vi "test_MSS SimulatedScope SimulatedFGen on ref in parallel.vi"(8 "Error In":errorcluster) -> (0 "Error Out":errorcluster)   [LabVIEW 2023]
uses:
  Measure and Stimulus Subsystems/Measure and Stimulus Subsystems.lvclass
panel:
  out "time":dbl
  out "Photosensor Waveform Chart":waveform(dbl)(graph)
  in  "Stop":bool
  out "Powersensor Scalar":dbl
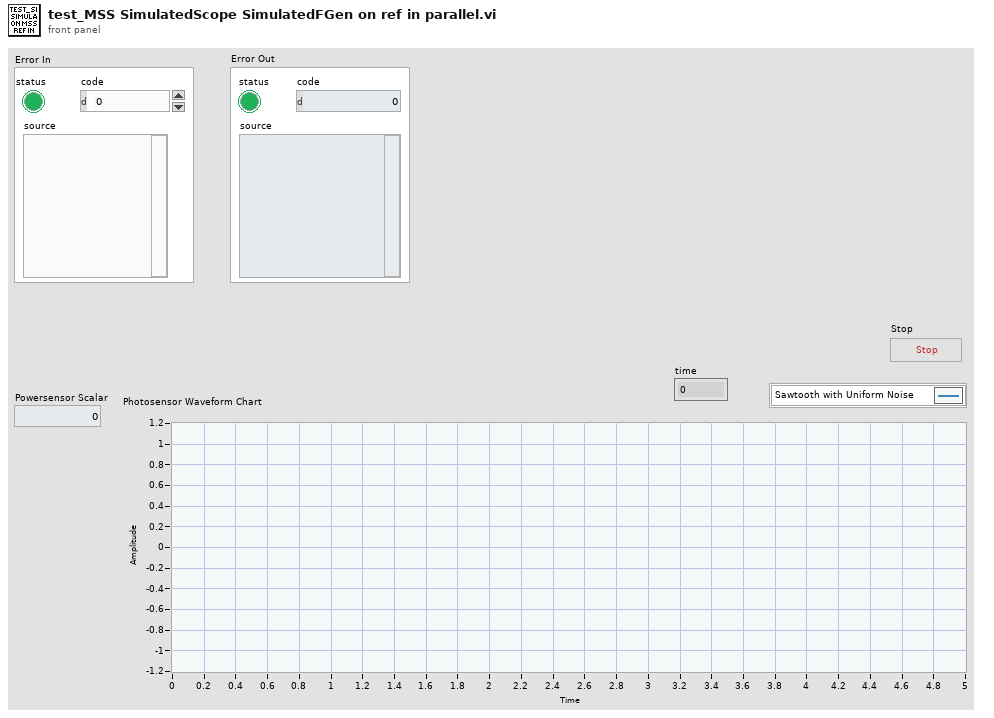
[diagram p1: front panel]
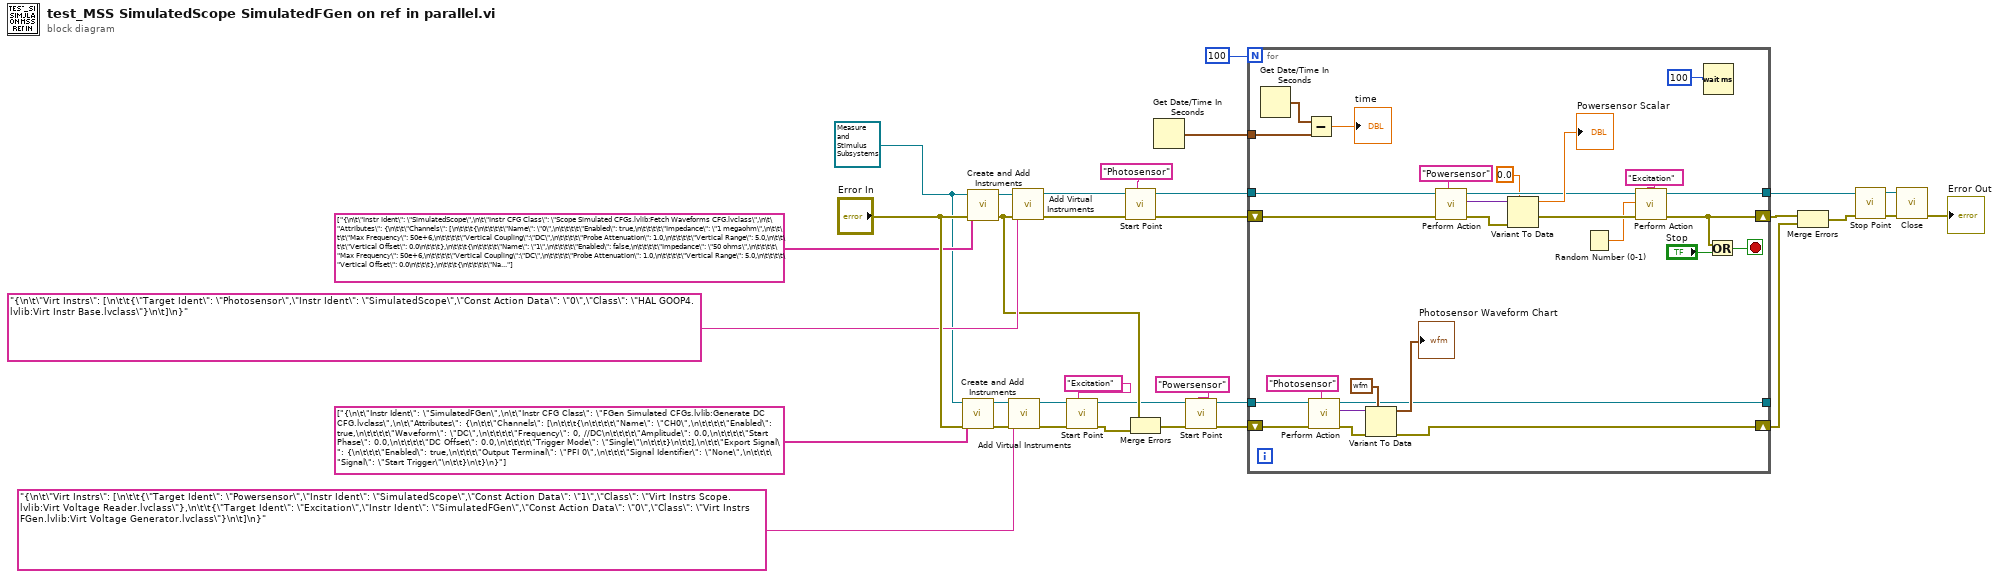
[diagram p0: block diagram]
diagram:
  w1 = refnum<class "Measure and Stimulus Subsystems.lvclass"> refnum ("MSS in")
  n1 = call "Create and Add Instruments.vi"("Error In"="Error In", "Physical Intr CFGs"=string[] ["{\n\t\"Instr Ident\": \"SimulatedFGen\",\n\t\"Instr CFG Class\": \"FGen Simulated CFGs.lvlib:Generate DC CFG.lvclass\",\n\t\"Attributes\": {\n\t\t\"Channels\": [\n\t\t\t{\n\t\t\t\t\"Name\": \"CH0\",\n\t\t\t\t\"Enabled\": true,\n\t\t\t\t\"Waveform\": \"DC\",\n\t\t\t\t\"Frequency\": 0, //DC\n\t\t\t\t\"Amplitude\": 0.0,\n\t\t\t\t\"Start Phase\": 0.0,\n\t\t\t\t\"DC Offset\": 0.0,\n\t\t\t\t\"Trigger Mode\": \"Single\"\n\t\t\t}\n\t\t],\n\t\t\"Export Signal\": {\n\t\t\t\"Enabled\": true,\n\t\t\t\"Output Terminal\": \"PFI 0\",\n\t\t\t\"Signal Identifier\": \"None\",\n\t\t\t\"Signal\": \"Start Trigger\"\n\t\t}\n\t}\n}"], "MSS in"=w1) -> ("Error Out"=w17:errorcluster, "MSS out"=w16:refnum<class "Measure and Stimulus Subsystems.lvclass">)  [unwired: 7 in]
  n2 = call "Create and Add Instruments.vi"("Error In"="Error In", "Physical Intr CFGs"=string[] ["{\n\t\"Instr Ident\": \"SimulatedScope\",\n\t\"Instr CFG Class\": \"Scope Simulated CFGs.lvlib:Fetch Waveforms CFG.lvclass\",\n\t\"Attributes\": {\n\t\t\"Channels\": [\n\t\t\t{\n\t\t\t\t\"Name\": \"0\",\n\t\t\t\t\"Enabled\": true,\n\t\t\t\t\"Impedance\": \"1 megaohm\",\n\t\t\t\t\"Max Frequency\": 50e+6,\n\t\t\t\t\"Vertical Coupling\":\"DC\",\n\t\t\t\t\"Probe Attenuation\": 1.0,\n\t\t\t\t\"Vertical Range\": 5.0,\n\t\t\t\t\"Vertical Offset\": 0.0\n\t\t\t},\n\t\t\t{\n\t\t\t\t\"Name\": \"1\",\n\t\t\t\t\"Enabled\": false,\n\t\t\t\t\"Impedance\": \"50 ohms\",\n\t\t\t\t\"Max Frequency\": 50e+6,\n\t\t\t\t\"Vertical Coupling\":\"DC\",\n\t\t\t\t\"Probe Attenuation\": 1.0,\n\t\t\t\t\"Vertical Range\": 5.0,\n\t\t\t\t\"Vertical Offset\": 0.0\n\t\t\t},\n\t\t\t{\n\t\t\t\t\"Name\": \"2\",\n\t\t\t\t\"Enabled\": false,\n\t\t\t\t\"Impedance\": \"50 ohms\",\n\t\t\t\t\"Max Frequency\": 50e+6,\n\t\t\t\t\"Vertical Coupling\":\"DC\",\n\t\t\t\t\"Probe Attenuation\": 1.0,\n\t\t\t\t\"Vertical Range\": 5.0,\n\t\t\t\t\"Vertical Offset\": 0.0\n\t\t\t},\n\t\t\t{\n\t\t\t\t\"Name\": \"3\",\n\t\t\t\t\"Enabled\": true,\n\t\t\t\t\"Impedance\": \"50 ohms\",\n\t\t\t\t\"Max Frequency\": 50e+6,\n\t\t\t\t\"Vertical Coupling\":\"DC\",\n\t\t\t\t\"Probe Attenuation\": 1.0,\n\t\t\t\t\"Vertical Range\": 1.4,\n\t\t\t\t\"Vertical Offset\": 0.0\n\t\t\t},\n\t\t\t{\n\t\t\t\t\"Name\": \"4\",\n\t\t\t\t\"Enabled\": false,\n\t\t\t\t\"Impedance\": \"50 ohms\",\n\t\t\t\t\"Max Frequency\": 50e+6,\n\t\t\t\t\"Vertical Coupling\":\"DC\",\n\t\t\t\t\"Probe Attenuation\": 1.0,\n\t\t\t\t\"Vertical Range\": 5.0,\n\t\t\t\t\"Vertical Offset\": 0.0\n\t\t\t},\n\t\t\t{\n\t\t\t\t\"Name\": \"5\",\n\t\t\t\t\"Enabled\": false,\n\t\t\t\t\"Impedance\": \"50 ohms\",\n\t\t\t\t\"Max Frequency\": 50e+6,\n\t\t\t\t\"Vertical Coupling\":\"DC\",\n\t\t\t\t\"Probe Attenuation\": 1.0,\n\t\t\t\t\"Vertical Range\": 5.0,\n\t\t\t\t\"Vertical Offset\": 0.0\n\t\t\t},\n\t\t\t{\n\t\t\t\t\"Name\": \"6\",\n\t\t\t\t\"Enabled\": false,\n\t\t\t\t\"Impedance\": \"50 ohms\",\n\t\t\t\t\"Max Frequency\": 50e+6,\n\t\t\t\t\"Vertical Coupling\":\"DC\",\n\t\t\t\t\"Probe Attenuation\": 1.0,\n\t\t\t\t\"Vertical Range\": 5.0,\n\t\t\t\t\"Vertical Offset\": 0.0\n\t\t\t},\n\t\t\t{\n\t\t\t\t\"Name\": \"7\",\n\t\t\t\t\"Enabled\": false,\n\t\t\t\t\"Impedance\": \"50 ohms\",\n\t\t\t\t\"Max Frequency\": 50e+6,\n\t\t\t\t\"Vertical Coupling\":\"DC\",\n\t\t\t\t\"Probe Attenuation\": 1.0,\n\t\t\t\t\"Vertical Range\": 5.0,\n\t\t\t\t\"Vertical Offset\": 0.0\n\t\t\t}\n\t\t],\n\t\t\"Horizontal\": {\n\t\t\t\"Enforce Realtime\": true,\n\t\t\t\"Number of Records\": 1,\n\t\t\t\"Min Sample Rate\": 1e+5,\n\t\t\t\"Reference Position\":50, //percent\n\t\t\t\"Min Record Length\":1e+3\n\t\t},\n\t\t\"Acquire\": {\n\t\t\t\"Type\": \"Normal\",\n\t\t\t\"NumSamples\": 1e+3,\n\t\t\t\"Fetch Relative To\": \"Read Pointer\"\n\t\t},\n\t\t\"Export Signal\": {\n\t\t\t\"Signal Identifier\": \"None\",\n\t\t\t\"Signal\": \"None\",\n\t\t\t\"Output Terminal\": \"None\"\n\t\t},\n\t\t\"Trigger\": {\n\t\t\t\"Type\": \"Immediate\",\n\t\t\t\"Slope\": \"Positive\",\n\t\t\t\"Source\": \"RTSI 0\",\n\t\t\t\"Holdoff\": 0.0,\n\t\t\t\"Delay\": 0.0\n\t\t}\n\t}\n}"], "MSS in"=w1) -> ("Error Out"=w9:errorcluster, "MSS out"=w21:refnum<class "Measure and Stimulus Subsystems.lvclass">)  [unwired: 7 in]
  n3 = call "Add Virtual Instruments.vi"("error in"=w17, "<JSON CFG>"="{\n\t\"Virt Instrs\": [\n\t\t{\"Target Ident\": \"Powersensor\",\"Instr Ident\": \"SimulatedScope\",\"Const Action Data\": \"1\",\"Class\": \"Virt Instrs Scope.lvlib:Virt Voltage Reader.lvclass\"},\n\t\t{\"Target Ident\": \"Excitation\",\"Instr Ident\": \"SimulatedFGen\",\"Const Action Data\": \"0\",\"Class\": \"Virt Instrs FGen.lvlib:Virt Voltage Generator.lvclass\"}\n\t]\n}", "MSS in"=w16) -> ("error out"=w11:errorcluster, "MSS out"=w12:refnum<class "Measure and Stimulus Subsystems.lvclass">)  [unwired: 7 in]
  n4 = call "Add Virtual Instruments.vi"("error in"=w9, "<JSON CFG>"="{\n\t\"Virt Instrs\": [\n\t\t{\"Target Ident\": \"Photosensor\",\"Instr Ident\": \"SimulatedScope\",\"Const Action Data\": \"0\",\"Class\": \"HAL GOOP4.lvlib:Virt Instr Base.lvclass\"}\n\t]\n}", "MSS in"=w21) -> ("error out"=w22:errorcluster, "MSS out"=w20:refnum<class "Measure and Stimulus Subsystems.lvclass">)  [unwired: 7 in]
  n5 = call "Start Point.vi"("Point Ident"="Excitation" ("Target Ident"), "error in"=w11, "MSS in"=w12) -> ("error out"=w8:errorcluster, "MSS out"=w7:refnum<class "Measure and Stimulus Subsystems.lvclass">)  [unwired: 7 in]
  n6 = call "Start Point.vi"("Point Ident"="Photosensor" ("Target Identifier"), "error in"=w22, "MSS in"=w20) -> ("error out"=w14:errorcluster, "MSS out"=w25:refnum<class "Measure and Stimulus Subsystems.lvclass">)  [unwired: 7 in]
  n7 = Merge Errors(w9, w8) -> (w10:errorcluster)
  n8 = Get Date/Time In Seconds() -> (seconds since 1Jan1904=w2:timestamp)
  n9 = call "Start Point.vi"("Point Ident"="Powersensor" ("Target Identifier"), "error in"=w10, "MSS in"=w7) -> ("error out"=w5:errorcluster, "MSS out"=w6:refnum<class "Measure and Stimulus Subsystems.lvclass">)  [unwired: 7 in]
  n10 = for {
    N: 100 -> [_]
    shift-right: [w55] -> w29
    shift-left: w14 -> [w61]
    tunnel: w6 -> [w45]
    shift-right: [w43] -> w3
    shift-left: w5 -> [w44]
    tunnel: [w42] -> _
    tunnel: w25 -> [w60]
    tunnel: [w53] -> w32
    tunnel: w2 -> [w41]
    stop <- w56 stop-if-true
    n11 = Get Date/Time In Seconds() -> (seconds since 1Jan1904=w40:timestamp)
    n12 = Subtract(x=w40, y=w41) -> (x-y=→"time":dbl)
    n13 = call "Perform Action.vi"("Point Ident"="Photosensor" ("Target Identifier"), "error in"=w44, "MSS in"=w45) -> ("error out"=w47:errorcluster, "Output"=w48:variant, "MSS out"=w42:refnum<class "Measure and Stimulus Subsystems.lvclass">)  [unwired: 6 in]
    n14 = Variant To Data(error in=w47, type=waveform(dbl) {"t0"=timestamp(0 s since 1904-01-01), "dt"=1.0, "Y"=[]} ("Waveform"), Variant=w48) -> (data=→"Photosensor Waveform Chart":waveform(dbl), error out=w43:errorcluster)
    n15 = call "Perform Action.vi"("Point Ident"="Powersensor" ("Target Identifier"), "error in"=w61, "MSS in"=w60) -> ("error out"=w36:errorcluster, "Output"=w35:variant, "MSS out"=w54:refnum<class "Measure and Stimulus Subsystems.lvclass">)  [unwired: 6 in]
    n16 = Variant To Data(error in=w36, type=0.0, Variant=w35) -> (data=→"Powersensor Scalar":dbl, error out=w57:errorcluster)
    n17 = Random Number (0-1)() -> (number: 0 to 1=w51:dbl)
    n18 = call "Perform Action.vi"("Point Ident"="Excitation" ("Target Ident"), "error in"=w57, "Input"=w51, "MSS in"=w54) -> ("error out"=w55:errorcluster, "MSS out"=w53:refnum<class "Measure and Stimulus Subsystems.lvclass">)  [unwired: 5 in, 1 out]
    n19 = Wait (ms)(milliseconds to wait=u32 100) -> ()  [unwired: 1 out]
    n20 = Or(x=w55, y="Stop") -> (x .or. y?=w56:bool)
  }
  n21 = Merge Errors(w29, w3) -> (w4:errorcluster)
  n22 = call "Stop Point.vi"("error in"=w4, "MSS in"=w32) -> ("error out"=w33:errorcluster, "MSS out"=w31:refnum<class "Measure and Stimulus Subsystems.lvclass">)  [unwired: 8 in]
  n23 = call "Close.vi"("error in"=w33, "MSS in"=w31) -> ("error out"=→"Error Out":errorcluster)  [unwired: 8 in, 1 out]
